vi "Attacker.vi"(4 "balls":T3[](array[typedef]), 6 "geometry":T4, 9 "Opponent goalie":T1, 10 "Robot":T1, 11 "command\nenum":T5) -> (2 "output cluster":T1)   [LabVIEW 2016]
uses:
  Core/AI Robot.ctl
  Functions Enum.ctl
  Command Enum.ctl
  Core/Field Size.ctl
  Core/AI Ball.ctl
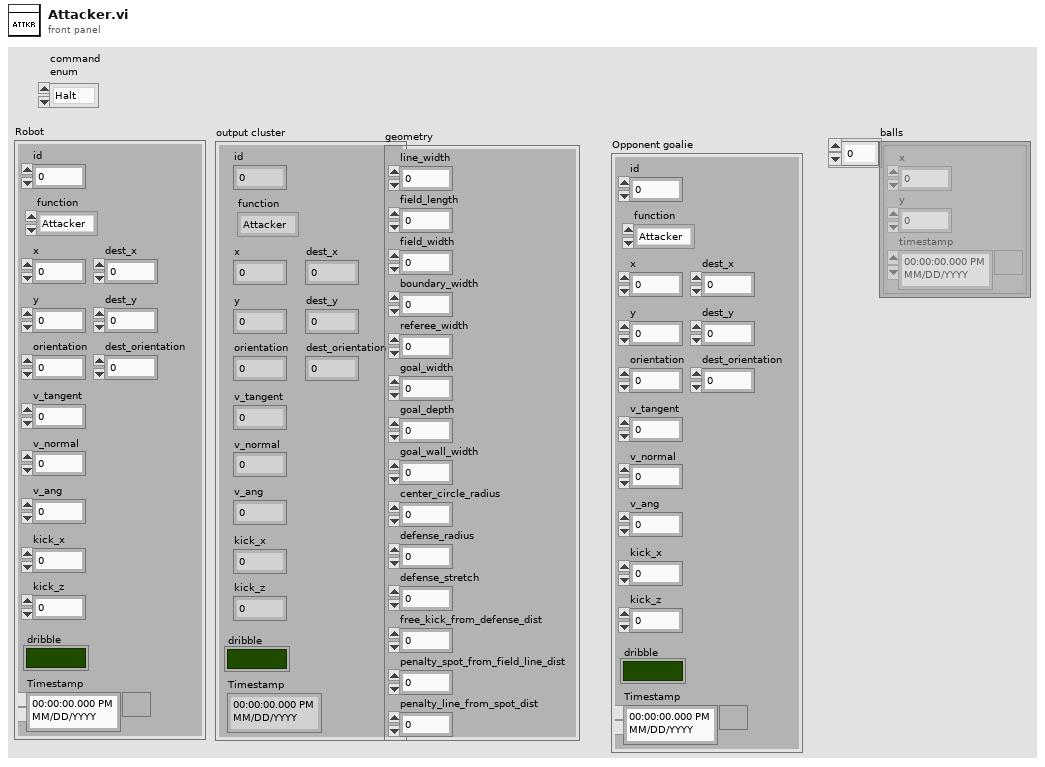
[diagram p1: front panel]
types:
  T1 = typedef "AI Robot.ctl" = cluster{"id":u32, "function":T2, "x":dbl, "y":dbl, "orientation":dbl, "v_tangent":dbl, "v_normal":dbl, "v_ang":dbl, "kick_x":dbl, "kick_z":dbl, "dribble":bool, "Timestamp":timestamp, "dest_x":dbl, "dest_y":dbl, "dest_orientation":dbl}
  T2 = typedef "Functions Enum.ctl" = enum16{"Attacker", "Goalie", "Defender", "Goto 0", "Dummy"}
  T3 = typedef "AI Ball.ctl" = cluster{"x":dbl, "y":dbl, "timestamp":timestamp}
  T4 = typedef "Field Size.ctl" = cluster{"line_width":u32, "field_length":u32, "field_width":u32, "boundary_width":u32, "referee_width":u32, "goal_width":u32, "goal_depth":u32, "goal_wall_width":u32, "center_circle_radius":u32, "defense_radius":u32, "defense_stretch":u32, "free_kick_from_defense_dist":u32, "penalty_spot_from_field_line_dist":u32, "penalty_line_from_spot_dist":u32}
  T5 = typedef "Command Enum.ctl" = enum16{"Halt", "Stop", "Force Start", "PKA Normal Start", "Prepare Kickoff Ally", "PKE Normal Start", "Prepare Kickoff Enemy", "Prepare Penalty Ally", "PPA Normal Start", "Prepare Penalty Enemy", "PPE Normal Start", "Direct Free Enemy", "Direct Free Ally", "Indirect Free Enemy", "Indirect Free Ally", "Timeout Enemy", "Timeout Ally", "Goal Enemy", "Goal Ally", "Ball Placement Enemy", "Ball Placement Ally", "None"}
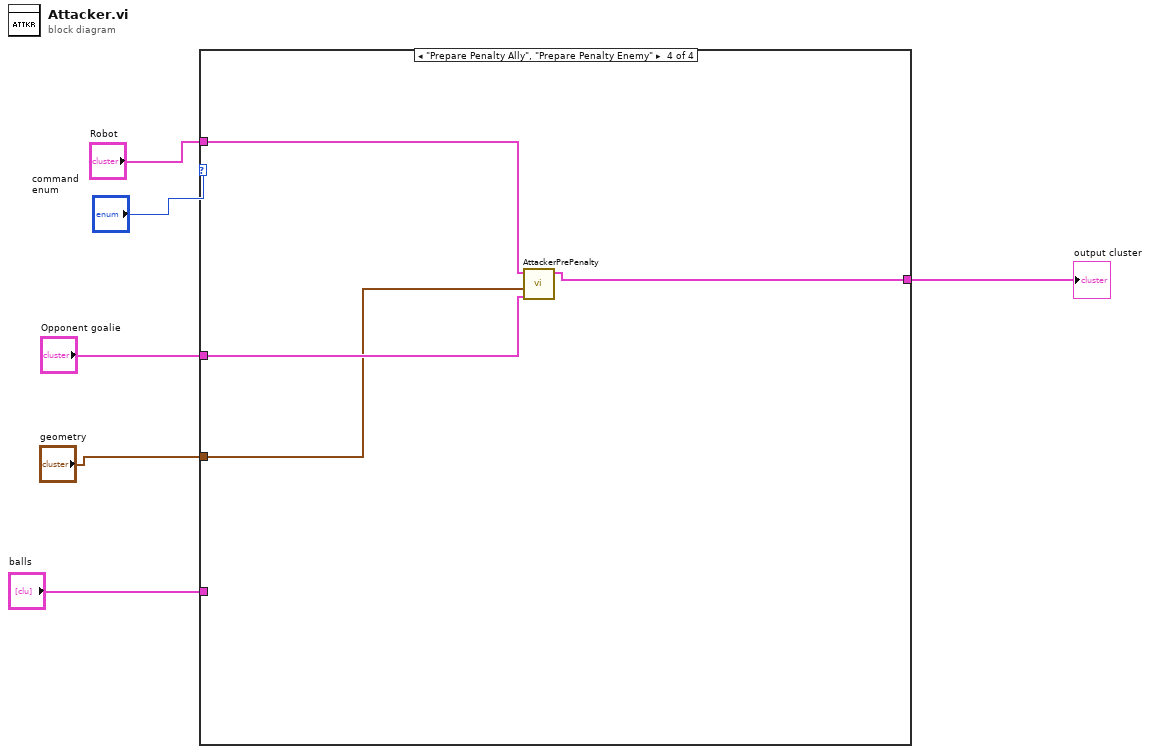
[diagram p0: block diagram]
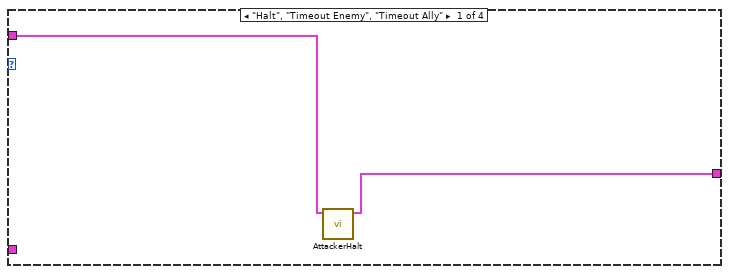
[diagram p2: hidden frame]
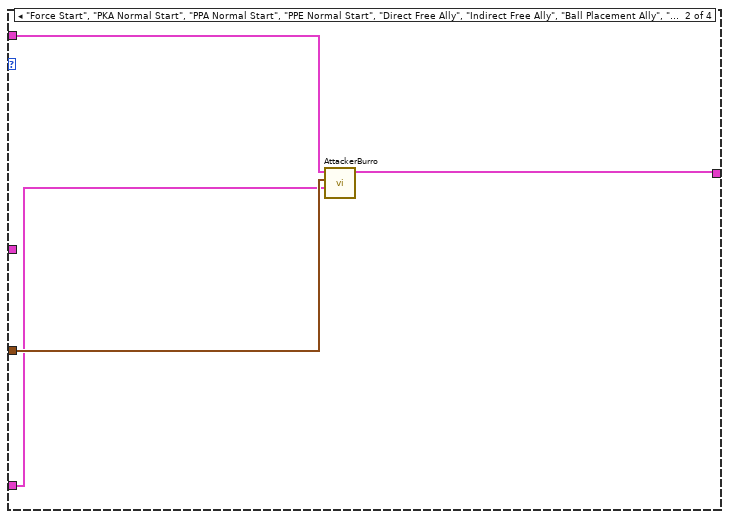
[diagram p3: hidden frame]
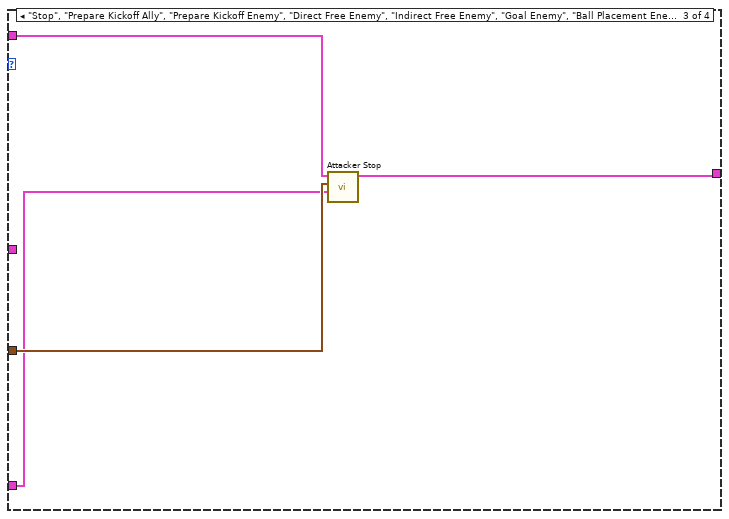
[diagram p4: hidden frame]
diagram:
  n1 = case shown="\"Prepare Penalty Ally\", \"Prepare Penalty Enemy\"" "command\nenum" {
    tunnel: "Robot" -> [w8 w12 w16 w19]
    tunnel: [w7 w9 w13 w17] -> w4
    tunnel: "Opponent goalie" -> [_ _ _ w20]
    tunnel: "geometry" -> [_ w11 w15 w18]
    tunnel: "balls" -> [_ w10 w14 _]
    frame "Halt", "Timeout Enemy", "Timeout Ally" {
      n2 = call "AttackerHalt.vi"("Robot in"=w8) -> ("Robot out"=w7:T1)  [unwired: 10 in]
    }
    frame "Force Start", "PKA Normal Start", "PPA Normal Start", "PPE Normal Start", "Direct Free Ally", "Indirect Free Ally", "Ball Placement Ally", "None", Default {
      n3 = call "AttackerBurro.vi"("balls"=w10, "Field Size in"=w11, "Robot in"=w12) -> ("Robot out"=w9:T1)  [unwired: 8 in]
    }
    frame "Stop", "Prepare Kickoff Ally", "Prepare Kickoff Enemy", "Direct Free Enemy", "Indirect Free Enemy", "Goal Enemy", "Ball Placement Enemy" {
      n4 = call "Attacker Stop.vi"("balls"=w14, "Field Size in"=w15, "Robot in"=w16) -> ("Robot out"=w13:T1)  [unwired: 8 in]
    }
    frame "Prepare Penalty Ally", "Prepare Penalty Enemy" {
      n5 = call "AttackerPrePenalty.vi"("Opponent goalie"=w20, "Field Size in"=w18, "Robot in"=w19) -> ("Robot out"=w17:T1)  [unwired: 8 in]
    }
  }
  "output cluster" <- w4
